vi "Get Scan Info for 藍芽.vi"(0 "String Input":string="$AGENT.81,C8.C8,S*03") -> (4 "MAC":string, 6 "ID":string, 8 "KPA":string, 10 "C":string, 14 "RSSI":string, 15 "V":string)   [LabVIEW 2019]
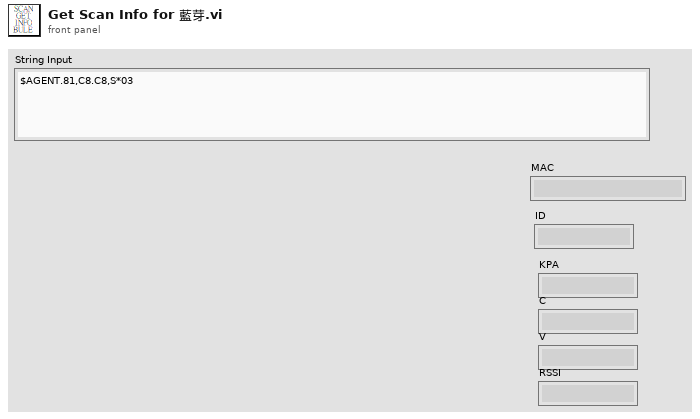
[diagram p1: front panel]
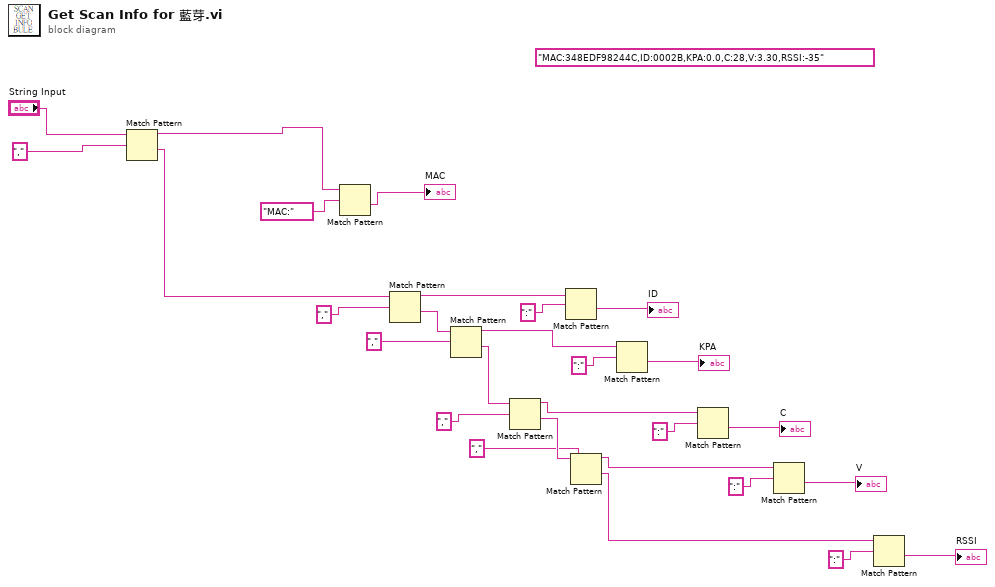
[diagram p0: block diagram]
diagram:
  (unwired) "MAC:348EDF98244C,ID:0002B,KPA:0.0,C:28,V:3.30,RSSI:-35"
  n1 = Match Pattern(string="String Input", regular expression=",") -> (before substring=w2:string, after substring=w3:string)  [unwired: 1 in, 2 out]
  n2 = Match Pattern(string=w2, regular expression="MAC:") -> (after substring=→"MAC":string)  [unwired: 1 in, 3 out]
  n3 = Match Pattern(string=w3, regular expression=",") -> (before substring=w19:string, after substring=w27:string)  [unwired: 1 in, 2 out]
  n4 = Match Pattern(string=w27, regular expression=",") -> (before substring=w14:string, after substring=w21:string)  [unwired: 1 in, 2 out]
  n5 = Match Pattern(string=w21, regular expression=",") -> (before substring=w11:string, after substring=w23:string)  [unwired: 1 in, 2 out]
  n6 = Match Pattern(string=w19, regular expression=":") -> (after substring=→"ID":string)  [unwired: 1 in, 3 out]
  n7 = Match Pattern(string=w23, regular expression=",") -> (before substring=w8:string, after substring=w5:string)  [unwired: 1 in, 2 out]
  n8 = Match Pattern(string=w14, regular expression=":") -> (after substring=→"KPA":string)  [unwired: 1 in, 3 out]
  n9 = Match Pattern(string=w11, regular expression=":") -> (after substring=→"C":string)  [unwired: 1 in, 3 out]
  n10 = Match Pattern(string=w8, regular expression=":") -> (after substring=→"V":string)  [unwired: 1 in, 3 out]
  n11 = Match Pattern(string=w5, regular expression=":") -> (after substring=→"RSSI":string)  [unwired: 1 in, 3 out]
